vi "ziGetValueString.vi"(3 "error in":errorcluster, 4 "Path":string, 5 "Handle In":T1 {"Handle" format="0x%08x"; "Conn" format="0x%08x"}) -> (0 "error out":errorcluster, 1 "Value":string, 2 "Handle Out":T1 {"Handle" format="0x%08x"; "Conn" format="0x%08x"})   [LabVIEW 2009, in "Zurich Instruments LabOne.lvlib"]
doc: "This vi retrieves the value of the node node specified by <b>Path</b> as a string <b>value</b>. The vi returns the value of the node first found if more than one node is available (a wildcard is used in <b>Path</b>). This function is only applicable to nodes that contain strings."
uses:
  <instrlib>/Zurich Instruments LabOne/Zurich Instruments LabOne.lvlib
  <instrlib>/Zurich Instruments LabOne/Public/ziTypeHandle.ctl
  <instrlib>/Zurich Instruments LabOne/Private/ziLV32.dll
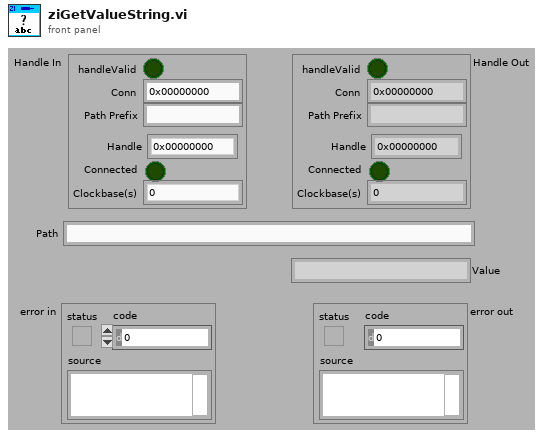
[diagram p1: front panel]
types:
  T1 = typedef "Zurich Instruments LabOne.lvlib/ziTypeHandle.ctl" = cluster{"handleValid":bool, "Conn":u64, "Path Prefix":string, "Handle":u64, "Connected":bool, "Clockbase(s)":dbl}
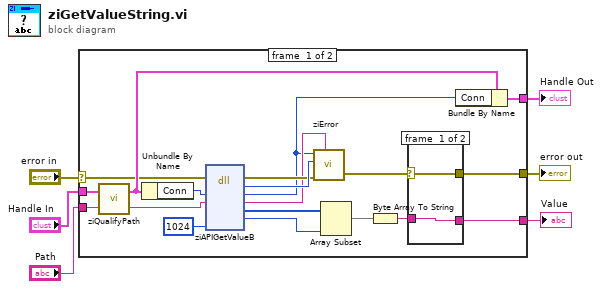
[diagram p0: block diagram]
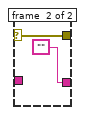
[diagram p2: hidden frame]
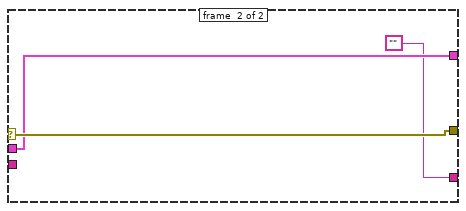
[diagram p3: hidden frame]
diagram:
  n1 = case shown="No Error" "error in" {
    selector: "error in" -> [w14 w32]
    tunnel: [w9 w32] -> w6
    tunnel: [w23 w31] -> w5
    tunnel: "Handle In" -> [w22 w31]
    tunnel: "Path" -> [w20 _]
    tunnel: [w7 ""] -> w2
    frame #0 {
      n2 = call <instrlib>:"ziQualifyPath.vi"("Path In"=w20, "Handle In"=w22) -> ("Path Out"=w19:string, "Handle Out"=w21:T1)
      n3 = Unbundle By Name(w21) -> ("Conn"=w12:u64)
      n4 = dll-call lib="C:/Program Files (x86)/National Instruments/LabVIEW 2009/instr.lib/Zurich Instruments LabOne/Private/ziLV*.*" fn="ziAPIGetValueB"(error in=w14, "Conn"=w12, "Path"=w19, "MaxLen"=1024) -> (error out=w24:errorcluster, "return type"=w25:u32, "Conn"=w11:u64, "Path"=w13:string, "Buffer"=w17:i8[], "Len"=w16:i32)  [unwired: 2 in, 4 out]
      n5 = call <instrlib>:"ziError.vi"("Conn"=w11, "ziErrorCode"=w25, "Error In"=w24, "Annotation"=w13) -> ("Error Out"=w10:errorcluster)  [unwired: 2 in]
      n6 = Array Subset(array=w17, length=w16) -> (w15:i8[])  [unwired: 1 in]
      n7 = Byte Array To String(unsigned byte array=w15) -> (string=w8:string)
      n8 = case shown="Error" w10 {
        selector: w10 -> [w27 w29]
        tunnel: [w27 w29] -> w9
        tunnel: w8 -> [w26 _]
        tunnel: [w26 ""] -> w7
        frame #0 {
        }
        frame #1 {
        }
      }
      n9 = Bundle By Name(cluster=w21, "Conn"=w11) -> (w23:T1)
    }
    frame #1 {
    }
  }
  "Handle Out" <- w5
  "error out" <- w6
  "Value" <- w2
